vi "Main - Pot.vi"() -> ()   [LabVIEW 2018]
uses:
  <vilib>/DAQmx/write.llb/DAQmx Write (Counter 1D Frequency NChan 1Samp).vi
  <vilib>/DAQmx/configure/timing.llb/DAQmx Timing (Implicit).vi
  <vilib>/DAQmx/read.llb/DAQmx Read (Analog DBL 1Chan 1Samp).vi
  typedef/Parametros control.ctl
  typedef/Selector control.ctl
panel:
  out "Tiempo de ciclo":u32
  out "Respuesta":cluster{"[0]":dbl, "[1]":dbl, "[2]":dbl}(graph)
  in  "Tipo de control":T1
  in  "Configuracion":T2={"Setpoint"=0.0, "Variable de proceso"=0.0, "Frecuencia PWM"=100.0, "Ciclo de trabajo PWM"=0.5000025, "V. histeresis (grados)"=0.0, "Ganacias PID"={"proportional gain (Kc)"=1.0, "integral time (Ti, min)"=inf, "derivative time (Td, min)"=0.0}} {"Variable de proceso" min=2.5e-06 max=1.0 step=0.1; "V. histeresis (grados)" min=2.5e-06 step=0.01}
  in  "Setpoint":dbl(knob) scale=-120.0..120.0
  out "Variable de proceso":dbl(knob) scale=-135.0..135.0
  in  "stop":bool
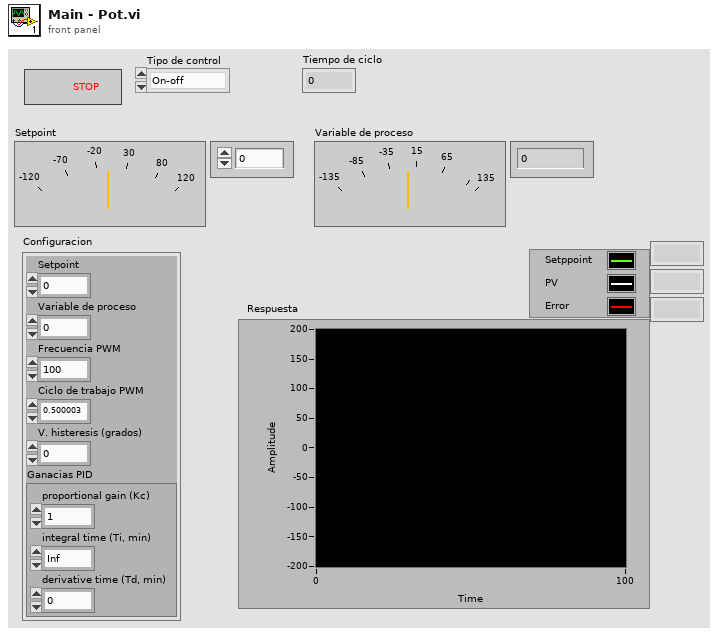
[diagram p1: front panel]
types:
  T1 = typedef "Selector control.ctl" = enum16{"On-off", "On-off hist.", "PID"}
  T2 = typedef "Parametros control.ctl" = cluster{"Setpoint":dbl, "Variable de proceso":dbl, "Frecuencia PWM":dbl, "Ciclo de trabajo PWM":dbl, "V. histeresis (grados)":dbl, "Ganacias PID":cluster{"proportional gain (Kc)":dbl, "integral time (Ti, min)":dbl, "derivative time (Td, min)":dbl}}
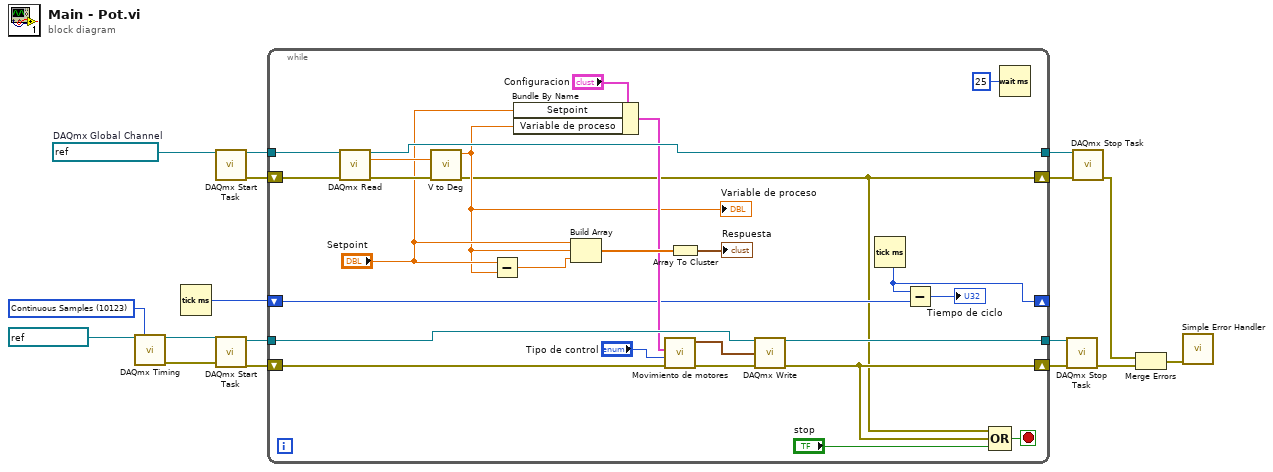
[diagram p0: block diagram]
diagram:
  w1 = refnum<k21> "Potenciometer"  # DAQmx Global Channel
  w9 = 10123 items=["Finite Samples"=10178, "Continuous Samples"=10123, "Hardware Timed Single Point"=12522] ("sample mode")
  n1 = call-poly <vilib>:"DAQmx Timing.vi"("task/channels in"=refnum<k21> "CW, CCW", "sample mode"=w9) -> ("task out"=w11:refnum<k21>, "error out"=w10:errorcluster)  [unwired: 12 in]
  n2 = Tick Count (ms)() -> (millisecond timer value=w3:u32)
  n3 = call <vilib>:"DAQmx Start Task.vi"("task/channels in"=w1) -> ("task out"=w17:refnum<k21>, "error out"=w16:errorcluster)  [unwired: 13 in]
  n4 = call <vilib>:"DAQmx Start Task.vi"("task/channels in"=w11, "error in"=w10) -> ("task out"=w13:refnum<k21>, "error out"=w12:errorcluster)  [unwired: 12 in]
  n5 = while {
    tunnel: w17 -> [w43]
    tunnel: [w39] -> w14
    tunnel: w13 -> [w37]
    tunnel: [w33] -> w7
    shift-right: [w21] -> _
    shift-left: w3 -> [w23]
    shift-right: [w18] -> w15
    shift-left: w16 -> [w41]
    shift-right: [w34] -> w8
    shift-left: w12 -> [w20]
    stop <- w35 stop-if-true
    n6 = call-poly <vilib>:"DAQmx Read.vi"("task/channels in"=w43, "error in"=w41) -> ("task out"=w39:refnum<k21>, "data"=w38:dbl, "error out"=w40:errorcluster)  [unwired: 11 in]
    n7 = call "V to Deg.vi"("Voltaje de entrada (0-5V)"=w38, "error in (no error)"=w40) -> ("Angulo [-135, 135]"=w24:dbl, "error out"=w18:errorcluster)  [unwired: 7 in]
    "Variable de proceso" <- w24
    n8 = Subtract(x="Setpoint", y=w24) -> (x-y=w29:dbl)
    n9 = Bundle By Name(cluster="Configuracion", "Setpoint"="Setpoint", "Variable de proceso"=w24) -> (w25:T2)
    n10 = Build Array("Setpoint", w24, w29) -> (w31:dbl[])
    n11 = call "Movimiento de motores.vi"("error in (no error)"=w20, "Tipo de control"="Tipo de control", "Parametros de control"=w25) -> ("error out"=w19:errorcluster, "Salida a motores"=w36:cluster{"duty cycle":dbl, "frequency":dbl}[])  [unwired: 7 in]
    n12 = Array To Cluster(array=w31) -> (cluster=→"Respuesta":cluster{"[0]":dbl, "[1]":dbl, "[2]":dbl})
    n13 = call-poly <vilib>:"DAQmx Write.vi"("task/channels in"=w37, "data"=w36, "error in"=w19) -> ("task out"=w33:refnum<k21>, "error out"=w34:errorcluster)  [unwired: 10 in, 1 out]
    n14 = Tick Count (ms)() -> (millisecond timer value=w21:u32)
    n15 = Subtract(x=w21, y=w23) -> (x-y=→"Tiempo de ciclo":u32)
    n16 = Compound Arithmetic op=OR(w18, w34, "stop") -> (w35:bool)
    n17 = Wait (ms)(milliseconds to wait=u32 25) -> ()  [unwired: 1 out]
  }
  n18 = call <vilib>:"DAQmx Stop Task.vi"("task/channels in"=w7, "error in"=w8) -> ("error out"=w6:errorcluster)  [unwired: 12 in, 1 out]
  n19 = call <vilib>:"DAQmx Stop Task.vi"("task/channels in"=w14, "error in"=w15) -> ("error out"=w5:errorcluster)  [unwired: 12 in, 1 out]
  n20 = Merge Errors(w5, w6) -> (w4:errorcluster)
  n21 = call <vilib>:"Simple Error Handler.vi"("error in (no error)"=w4) -> ()  [unwired: 4 in, 5 out]
